vi "IDS_displacement_linProc.vi"(0 "deviceHandle":i32, 1 "axis":i32, 2 "set":i32, 3 "fringesNbr":i32, 4 "samplesPerFringe":i32, 5 "error in (no error)":errorcluster) -> (14 "deviceHandle out":i32, 16 "linTable":dbl, 17 "nonLinearAmpl":dbl, 19 "error out":errorcluster)   [LabVIEW 2016]
doc: "int IDS_DLL IDS_ecu_enable();"
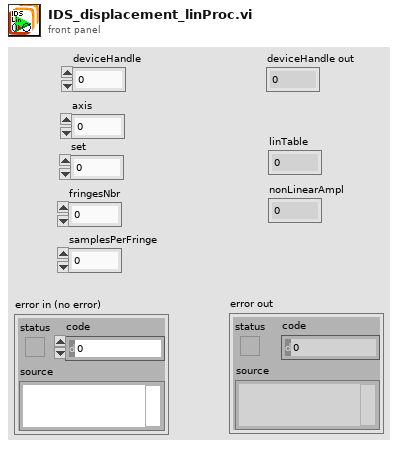
[diagram p1: front panel]
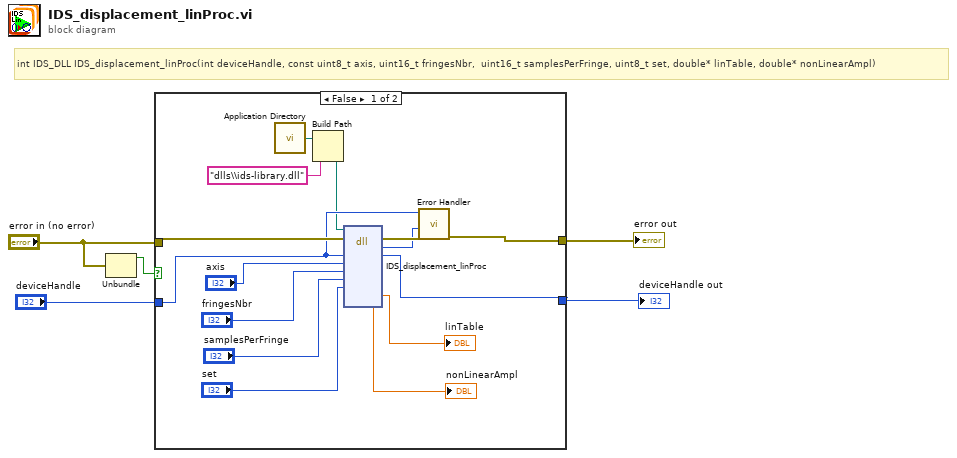
[diagram p0: block diagram]
diagram:
  # "int IDS_DLL IDS_displacement_linProc(int deviceHandle, const uint8_t axis, uint16_t fringesNbr,  uint16_t samplesPerFringe, uint8_t set, double* linTable, double* nonLinearAmpl)"
  n1 = Unbundle("error in (no error)") -> ("status"=w1:bool)  [unwired: 2 out]
  n2 = case shown="False" w1 {
    tunnel: "error in (no error)" -> [w20 w22]
    tunnel: [w18 w22] -> w5
    tunnel: "deviceHandle" -> [w12 w21]
    tunnel: [w17 w21] -> w3
    frame False {
      n3 = call <vilib>:"Application Directory.vi"() -> ("Application Directory"=w8:path)
      n4 = Build Path(base path=w8, name or relative path="dlls\\ids-library.dll" ("ipAddress")) -> (appended path=w6:path)
      n5 = dll-call lib="C:/Users/matheus/Desktop/LabVIEW_Draft_V1.6.0/dlls/ids-library.*" fn="IDS_displacement_linProc"(path in=w6, error in=w20, "deviceHandle"=w12, "axis"="axis", "fringesNbr"="fringesNbr", "samplesPerFringe"="samplesPerFringe", "set"="set") -> (error out=w19:errorcluster, "return type"=w16:i32, "deviceHandle"=w17:i32, "linTable"=→"linTable":dbl, "nonLinearAmpl"=→"nonLinearAmpl":dbl)  [unwired: 7 in, 1 out]
      n6 = call "Error Handler.vi"("error in (no error)"=w19, "error code"=w16, "deviceHandle"=w12) -> ("error out"=w18:errorcluster)  [unwired: 7 in, 1 out]
    }
    frame True {
    }
  }
  "error out" <- w5
  "deviceHandle out" <- w3
